vi "Move for TimeVelocity.vi"(6 "Wheel DevRef":T2[](array[typedef])=[{"DeviceStatus"={"status"=FALSE, "code"=0, "source"=""}, "Type"=enum."CAN", "PWM"={"PWM Channel"=enum."PWM 1", "DeadBand"={"Name"="", "maxPositivePwm"=0, "minPositivePwm"=0, "centerPwm"=0, "maxNegativePwm"=0, "minNegativePwm"=0, "angularRange"=0}}, "CAN"={"Device Number"=3, "SetOutput VI Ref"=variant(refnum<vi> refnum), "GetOutput VI Ref"=variant(refnum<vi> refnum), "Enable VI Ref"=variant(refnum<vi> refnum), "Disable VI Ref"=variant(refnum<vi> refnum), "Data"=variant(cluster{"Control Mode":enum8{"Percent VBus", "Speed", "Position", "Slave", "Unchanged / Invalid", "Voltage Compensation", "Current", "Motion Profile", "Motion Magic"}, "Encoder Initial Position":dbl, "MaxVout":dbl} {"Control Mode"=enum."Percent VBus", "Encoder Initial Position"=0.0, "MaxVout"=12.0})}, "Invert"=TRUE}, {"DeviceStatus"={"status"=FALSE, "code"=0, "source"=""}, "Type"=enum."CAN", "PWM"={"PWM Channel"=enum."PWM 1", "DeadBand"={"Name"="", "maxPositivePwm"=0, "minPositivePwm"=0, "centerPwm"=0, "maxNegativePwm"=0, "minNegativePwm"=0, "angularRange"=0}}, "CAN"={"Device Number"=7, "SetOutput VI Ref"=variant(refnum<vi> refnum), "GetOutput VI Ref"=variant(refnum<vi> refnum), "Enable VI Ref"=variant(refnum<vi> refnum), "Disable VI Ref"=variant(refnum<vi> refnum), "Data"=variant(cluster{"Control Mode":enum8{"Percent VBus", "Speed", "Position", "Slave", "Unchanged / Invalid", "Voltage Compensation", "Current", "Motion Profile", "Motion Magic"}, "Encoder Initial Position":dbl, "MaxVout":dbl} {"Control Mode"=enum."Percent VBus", "Encoder Initial Position"=0.0, "MaxVout"=12.0})}, "Invert"=TRUE}, {"DeviceStatus"={"status"=FALSE, "code"=0, "source"=""}, "Type"=enum."CAN", "PWM"={"PWM Channel"=enum."PWM 1", "DeadBand"={"Name"="", "maxPositivePwm"=0, "minPositivePwm"=0, "centerPwm"=0, "maxNegativePwm"=0, "minNegativePwm"=0, "angularRange"=0}}, "CAN"={"Device Number"=5, "SetOutput VI Ref"=variant(refnum<vi> refnum), "GetOutput VI Ref"=variant(refnum<vi> refnum), "Enable VI Ref"=variant(refnum<vi> refnum), "Disable VI Ref"=variant(refnum<vi> refnum), "Data"=variant(cluster{"Control Mode":enum8{"Percent VBus", "Speed", "Position", "Slave", "Unchanged / Invalid", "Voltage Compensation", "Current", "Motion Profile", "Motion Magic"}, "Encoder Initial Position":dbl, "MaxVout":dbl} {"Control Mode"=enum."Percent VBus", "Encoder Initial Position"=0.0, "MaxVout"=12.0})}, "Invert"=FALSE}, {"DeviceStatus"={"status"=FALSE, "code"=0, "source"=""}, "Type"=enum."CAN", "PWM"={"PWM Channel"=enum."PWM 1", "DeadBand"={"Name"="", "maxPositivePwm"=0, "minPositivePwm"=0, "centerPwm"=0, "maxNegativePwm"=0, "minNegativePwm"=0, "angularRange"=0}}, "CAN"={"Device Number"=1, "SetOutput VI Ref"=variant(refnum<vi> refnum), "GetOutput VI Ref"=variant(refnum<vi> refnum), "Enable VI Ref"=variant(refnum<vi> refnum), "Disable VI Ref"=variant(refnum<vi> refnum), "Data"=variant(cluster{"Control Mode":enum8{"Percent VBus", "Speed", "Position", "Slave", "Unchanged / Invalid", "Voltage Compensation", "Current", "Motion Profile", "Motion Magic"}, "Encoder Initial Position":dbl, "MaxVout":dbl} {"Control Mode"=enum."Percent VBus", "Encoder Initial Position"=0.0, "MaxVout"=12.0})}, "Invert"=FALSE}], 7 "Swerve DevRef":T2[](array[typedef])=[{"DeviceStatus"={"status"=FALSE, "code"=0, "source"=""}, "Type"=enum."CAN", "PWM"={"PWM Channel"=enum."PWM 1", "DeadBand"={"Name"="", "maxPositivePwm"=0, "minPositivePwm"=0, "centerPwm"=0, "maxNegativePwm"=0, "minNegativePwm"=0, "angularRange"=0}}, "CAN"={"Device Number"=4, "SetOutput VI Ref"=variant(refnum<vi> refnum), "GetOutput VI Ref"=variant(refnum<vi> refnum), "Enable VI Ref"=variant(refnum<vi> refnum), "Disable VI Ref"=variant(refnum<vi> refnum), "Data"=variant(cluster{"Control Mode":enum8{"Percent VBus", "Speed", "Position", "Slave", "Unchanged / Invalid", "Voltage Compensation", "Current", "Motion Profile", "Motion Magic"}, "Encoder Initial Position":dbl, "MaxVout":dbl} {"Control Mode"=enum."Position", "Encoder Initial Position"=0.0, "MaxVout"=12.0})}, "Invert"=FALSE}, {"DeviceStatus"={"status"=FALSE, "code"=0, "source"=""}, "Type"=enum."CAN", "PWM"={"PWM Channel"=enum."PWM 1", "DeadBand"={"Name"="", "maxPositivePwm"=0, "minPositivePwm"=0, "centerPwm"=0, "maxNegativePwm"=0, "minNegativePwm"=0, "angularRange"=0}}, "CAN"={"Device Number"=8, "SetOutput VI Ref"=variant(refnum<vi> refnum), "GetOutput VI Ref"=variant(refnum<vi> refnum), "Enable VI Ref"=variant(refnum<vi> refnum), "Disable VI Ref"=variant(refnum<vi> refnum), "Data"=variant(cluster{"Control Mode":enum8{"Percent VBus", "Speed", "Position", "Slave", "Unchanged / Invalid", "Voltage Compensation", "Current", "Motion Profile", "Motion Magic"}, "Encoder Initial Position":dbl, "MaxVout":dbl} {"Control Mode"=enum."Position", "Encoder Initial Position"=0.0, "MaxVout"=12.0})}, "Invert"=FALSE}, {"DeviceStatus"={"status"=FALSE, "code"=0, "source"=""}, "Type"=enum."CAN", "PWM"={"PWM Channel"=enum."PWM 1", "DeadBand"={"Name"="", "maxPositivePwm"=0, "minPositivePwm"=0, "centerPwm"=0, "maxNegativePwm"=0, "minNegativePwm"=0, "angularRange"=0}}, "CAN"={"Device Number"=6, "SetOutput VI Ref"=variant(refnum<vi> refnum), "GetOutput VI Ref"=variant(refnum<vi> refnum), "Enable VI Ref"=variant(refnum<vi> refnum), "Disable VI Ref"=variant(refnum<vi> refnum), "Data"=variant(cluster{"Control Mode":enum8{"Percent VBus", "Speed", "Position", "Slave", "Unchanged / Invalid", "Voltage Compensation", "Current", "Motion Profile", "Motion Magic"}, "Encoder Initial Position":dbl, "MaxVout":dbl} {"Control Mode"=enum."Position", "Encoder Initial Position"=0.0, "MaxVout"=12.0})}, "Invert"=FALSE}, {"DeviceStatus"={"status"=FALSE, "code"=0, "source"=""}, "Type"=enum."CAN", "PWM"={"PWM Channel"=enum."PWM 1", "DeadBand"={"Name"="", "maxPositivePwm"=0, "minPositivePwm"=0, "centerPwm"=0, "maxNegativePwm"=0, "minNegativePwm"=0, "angularRange"=0}}, "CAN"={"Device Number"=2, "SetOutput VI Ref"=variant(refnum<vi> refnum), "GetOutput VI Ref"=variant(refnum<vi> refnum), "Enable VI Ref"=variant(refnum<vi> refnum), "Disable VI Ref"=variant(refnum<vi> refnum), "Data"=variant(cluster{"Control Mode":enum8{"Percent VBus", "Speed", "Position", "Slave", "Unchanged / Invalid", "Voltage Compensation", "Current", "Motion Profile", "Motion Magic"}, "Encoder Initial Position":dbl, "MaxVout":dbl} {"Control Mode"=enum."Position", "Encoder Initial Position"=0.0, "MaxVout"=12.0})}, "Invert"=FALSE}], 8 "error in":errorcluster, 9 "Motor Power":dbl, 10 "Drive Angle":dbl, 11 "Max Time":i32) -> (0 "error out":errorcluster)   [LabVIEW 2016]
uses:
  <vilib>/Rock Robotics/WPI/MotorControl/WPI_MotorControlDeviceRef.ctl
  <vilib>/Rock Robotics/WPI/MotorControl/WPI_MotorControlType.ctl
  <vilib>/Rock Robotics/SystemInterfaces/DIO/FPGA_DIOPWMChannel.ctl
  <vilib>/Rock Robotics/WPI/PWM/WPI_PWMDeadband.ctl
  <vilib>/addons/control/pid/pid.llb/PID (DBL).vi
  <vilib>/addons/control/pid/NI_PID_pid.lvlib
panel:
  out "PID Output":dbl(graph)
  out "Sensor Velocity":dbl(graph)
  out "Difference":dbl(graph)
  in  "output range":cluster{"output high":dbl, "output low":dbl}={"output high"=1.0, "output low"=-1.0} {"output low" format="%.2f"; "output high" format="%.2f"}
  in  "PID gains Rotational Correction":T1={"proportional gain (Kc)"=2.5e-05, "integral time (Ti, min)"=0.0, "derivative time (Td, min)"=0.0} {"derivative time (Td, min)" format="%.3f"; "integral time (Ti, min)" format="%.3f"; "proportional gain (Kc)" format="%.9f"}
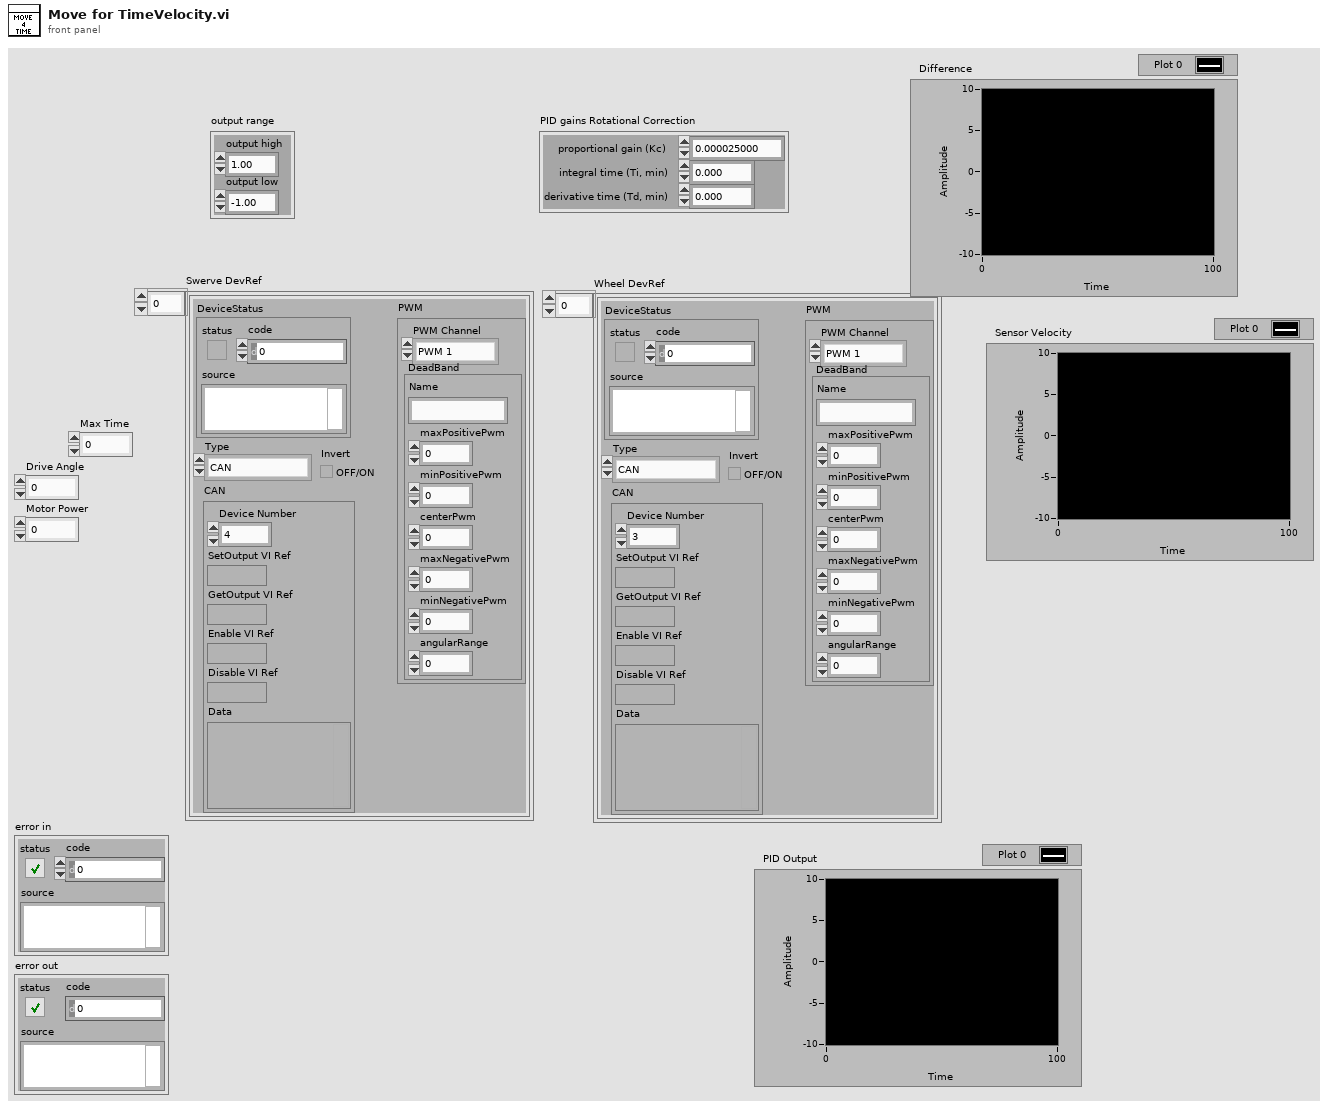
[diagram p1: front panel]
types:
  T1 = cluster{"proportional gain (Kc)":dbl, "integral time (Ti, min)":dbl, "derivative time (Td, min)":dbl}
  T2 = typedef "WPI_MotorControlDeviceRef.ctl" = cluster{"DeviceStatus":errorcluster, "Type":T3, "PWM":cluster{"PWM Channel":T4, "DeadBand":T5}, "CAN":cluster{"Device Number":u8, "SetOutput VI Ref":variant, "GetOutput VI Ref":variant, "Enable VI Ref":variant, "Disable VI Ref":variant, "Data":variant}, "Invert":bool}
  T3 = typedef "WPI_MotorControlType.ctl" = enum16{"PWM", "CAN"}
  T4 = typedef "FPGA_DIOPWMChannel.ctl" = enum8{"PWM 0", "PWM 1", "PWM 2", "PWM 3", "PWM 4", "PWM 5", "PWM 6", "PWM 7", "PWM 8", "PWM 9", "PWM MXP 0", "PWM MXP 1", "PWM MXP 2", "PWM MXP 3", "PWM MXP 4", "PWM MXP 5", "PWM MXP 6", "PWM MXP 7", "PWM MXP 8", "PWM MXP 9", "Invalid"}
  T5 = typedef "WPI_PWMDeadband.ctl" = cluster{"Name":string, "maxPositivePwm":i32, "minPositivePwm":i32, "centerPwm":i32, "maxNegativePwm":i32, "minNegativePwm":i32, "angularRange":u16}
  T6 = typedef "WPI_CANTalonSRX_GlobalStatus.ctl" = cluster{"Applied Throttle":dbl, "Module Enabled":bool, "CAN Error":errorcluster, "Closed Loop Error":dbl, "Forward Limit Switch Closed":bool, "Reverse Limit Switch Closed":bool, "Sensor Position":dbl, "Sensor Velocity":dbl, "Current":dbl, "Sticky Fault - Over Temp":bool, "Sticky Fault - Under Voltage":bool, "Sticky Fault - Forward Limit":bool, "Sticky Fault - Reverse Limit":bool, "Sticky Fault - Forward Soft Limit":bool, "Sticky Fault - Reverse Soft Limit":bool, "Brake is Enabled":bool, "Encoder Position":dbl, "Encoder Velocity":dbl, "Encoder Index Count":dbl, "Encoder A Pin State":bool, "Encoder B Pin State":bool, "Encoder Index Pin State":bool, "Analog In":dbl, "Analog In Velocity":dbl, "Temperature (C)":dbl, "Battery Voltage":dbl, "Control 5 Is Supported":bool, "Current Profile Slot Select":dbl, "Pos Div 8":bool, "Vel Div 4":bool, "Pulse Width Position":i32, "Pulse Width Velocity":i32, "Pulse Width Rise To Rise (us)":i32, "Pulse Width Rise To Fall (us)":i32, "Mot Prof Active Is Under Run":bool, "Mot Prof Active Has Under Run":bool, "Mot Prof Active Is Last":bool, "Mot Prof Active Velocity Only":bool, "Mot Prof Active Is Valid":bool, "Mot Prof Buffer Is Full":bool, "Mot Prof Active Profile Slot Select":i32, "Mot Prof NextID":i32, "Mot Prof Count":i32, "Mot Prof Active Velocity":dbl, "Mot Prof Active Position":dbl, "Mot Prof Output Enable":i32}
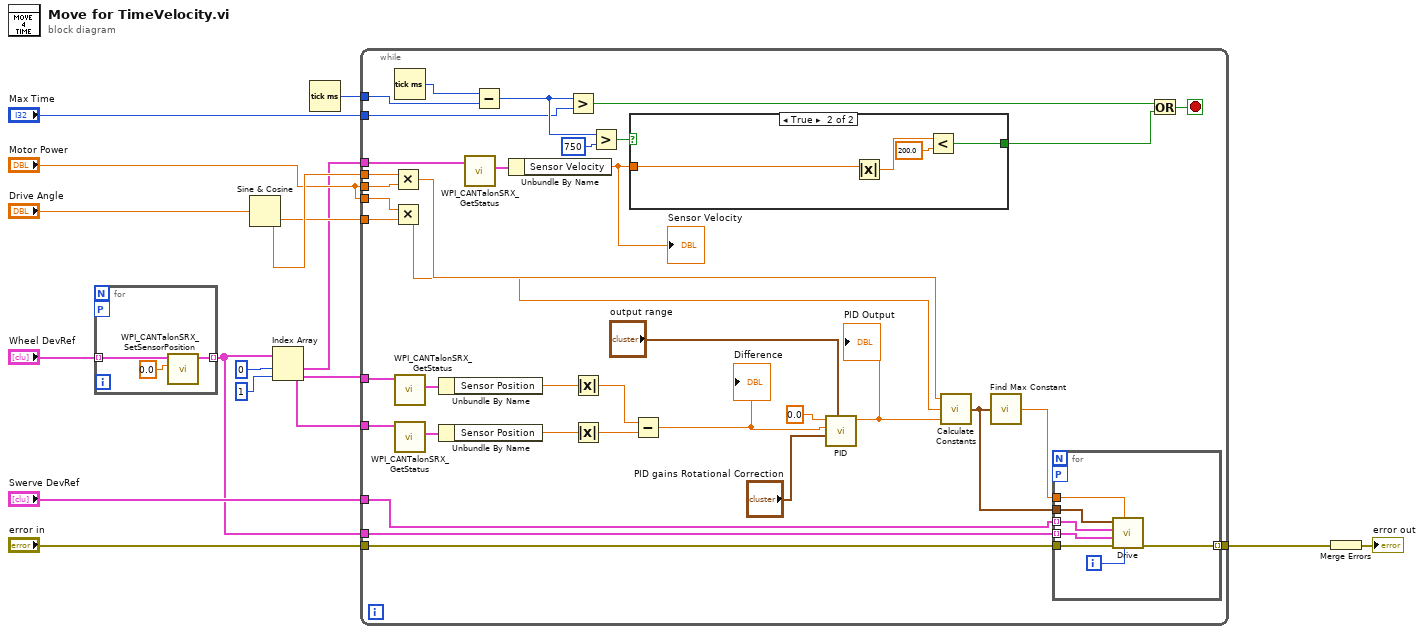
[diagram p0: block diagram]
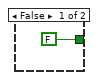
[diagram p2: hidden frame]
diagram:
  n1 = for {
    tunnel: "Wheel DevRef" -> [w19] mode=indexing
    tunnel: [w17] -> w7 mode=indexing
    workers-P: _ -> [_]
    n2 = call <vilib>:"WPI_CANTalonSRX_SetSensorPosition.vi"("New Sensor Position"=0.0, "CAN Talon SRX Ref"=w19) -> ("CAN Talon SRX Ref"=w17:T2)  [unwired: 8 in, 1 out]
  }
  n3 = Sine & Cosine(0:"Drive Angle") -> (1:w12:dbl, 2:w11:dbl)
  n4 = Index Array(array=w7, index #1=0 ("index"), index #2=1 ("index")) -> (element #1=w4:T2, element #2=w3:T2)
  n5 = Tick Count (ms)() -> (millisecond timer value=w9:u32)
  n6 = while {
    tunnel: "Swerve DevRef" -> [w54]
    tunnel: w7 -> [w53]
    tunnel: "error in" -> [w52]
    tunnel: w12 -> [w51]
    tunnel: "Motor Power" -> [w49]
    tunnel: w11 -> [w47]
    tunnel: "Motor Power" -> [w46]
    tunnel: w9 -> [w44]
    tunnel: "Max Time" -> [w41]
    tunnel: w4 -> [w21]
    tunnel: [w36] -> w6
    tunnel: w4 -> [w29]
    tunnel: w3 -> [w30]
    stop <- w37 stop-if-true
    n7 = Multiply(x=w51, y=w49) -> (x*y=w50:dbl)
    n8 = Multiply(x=w46, y=w47) -> (x*y=w48:dbl)
    n9 = Tick Count (ms)() -> (millisecond timer value=w45:u32)
    n10 = call <vilib>:"WPI_CANTalonSRX_GetStatus.vi"("CAN Talon SRX Ref"=w30) -> ("Talon SRX Status"=w32:T6)  [unwired: 8 in, 2 out]
    n11 = call <vilib>:"WPI_CANTalonSRX_GetStatus.vi"("CAN Talon SRX Ref"=w29) -> ("Talon SRX Status"=w31:T6)  [unwired: 8 in, 2 out]
    n12 = Unbundle By Name(w32) -> ("Sensor Position"=w28:dbl)
    n13 = Unbundle By Name(w31) -> ("Sensor Position"=w27:dbl)
    n14 = call <vilib>:"WPI_CANTalonSRX_GetStatus.vi"("CAN Talon SRX Ref"=w21) -> ("Talon SRX Status"=w22:T6)  [unwired: 8 in, 2 out]
    n15 = Subtract(x=w45, y=w44) -> (x-y=w42:u32)
    n16 = Unbundle By Name(w22) -> ("Sensor Velocity"=w20:dbl)
    "Sensor Velocity" <- w20
    n17 = Greater?(x=w42, y=w41) -> (0:w39:bool)
    n18 = Absolute Value(x=w28) -> (abs(x)=w25:dbl)
    n19 = Absolute Value(x=w27) -> (abs(x)=w26:dbl)
    n20 = Greater?(x=w42, y=u32 750) -> (0:w43:bool)
    n21 = case shown="True" w43 {
      tunnel: [FALSE w60] -> w38
      tunnel: w20 -> [_ w58]
      frame False {
      }
      frame True {
        n22 = Absolute Value(x=w58) -> (abs(x)=w59:dbl)
        n23 = Less?(x=w59, y=200.0) -> (x < y?=w60:bool)
      }
    }
    n24 = Subtract(x=w25, y=w26) -> (x-y=w24:dbl)
    "Difference" <- w24
    n25 = call-poly <vilib>:"PID.vi"("output range"="output range", "PID gains"="PID gains Rotational Correction", "process variable"=w24, "setpoint"=0.0) -> ("output"=w23:dbl)  [unwired: 6 in, 1 out]
    "PID Output" <- w23
    n26 = call "Calculate Constants.vi"("Z"=w23, "Y"=w48, "X"=w50) -> ("constants cluster"=w55:cluster{"a":dbl, "b":dbl, "c":dbl, "d":dbl})
    n27 = call "Find Max Constant.vi"("constants"=w55) -> ("Max or 1"=w56:dbl)
    n28 = for {
      tunnel: w55 -> [w68]
      tunnel: w54 -> [w67] mode=indexing
      tunnel: w53 -> [w66] mode=indexing
      workers-P: _ -> [_]
      tunnel: [w64] -> w36 mode=indexing
      tunnel: w52 -> [w63]
      tunnel: w56 -> [w62]
      i -> [w65]
      n29 = call "Drive.vi"("Index"=w65, "Max Speed or 1"=w62, "error in"=w63, "Wheel DevRef"=w66, "Swerve DevRef"=w67, "constants"=w68) -> ("error out"=w64:errorcluster)  [unwired: 1 in, 4 out]
    }
    n30 = Or(x=w39, y=w38) -> (x .or. y?=w37:bool)
  }
  n31 = Merge Errors(w6) -> (→"error out":errorcluster)
